vi "unpackWarn.vi"(6 "长度":i32, 7 "数据":u8[](array[numeric]) format="%.0x") -> (2 "告警状态":bool, 3 "告警信息":string)   [LabVIEW 2014]
panel:
  out "告警信息":string
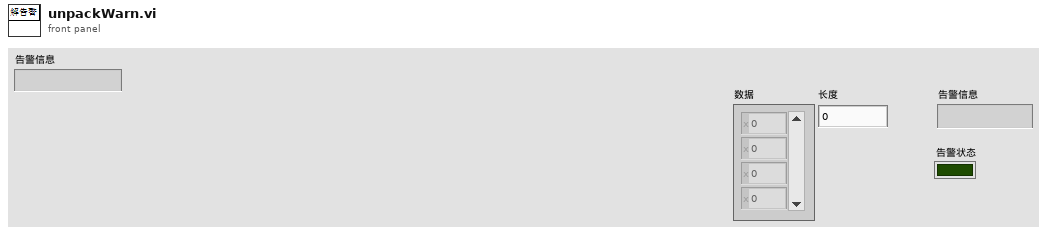
[diagram p1: front panel]
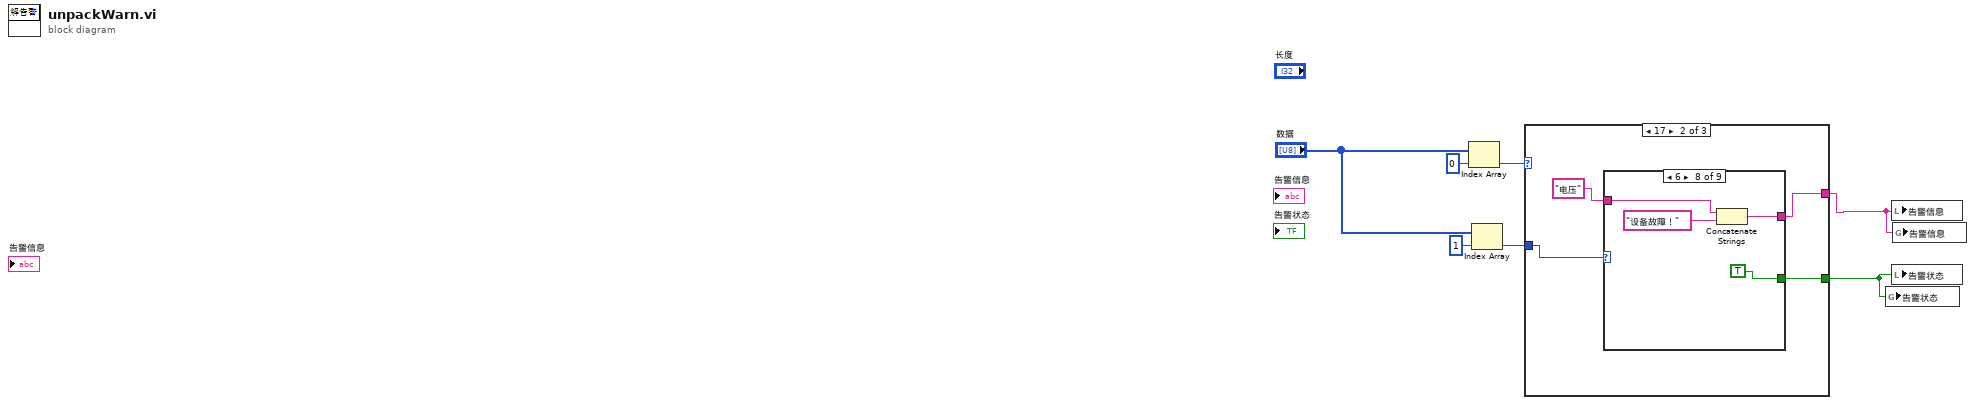
[diagram p0: block diagram]
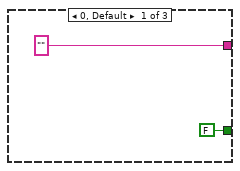
[diagram p2: hidden frame]
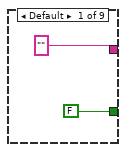
[diagram p3: hidden frame]
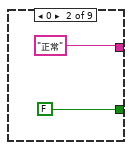
[diagram p4: hidden frame]
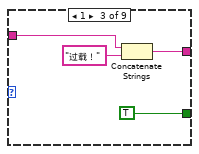
[diagram p5: hidden frame]
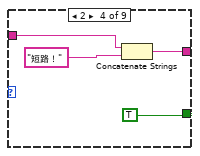
[diagram p6: hidden frame]
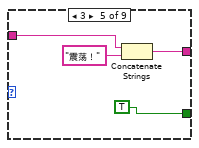
[diagram p7: hidden frame]
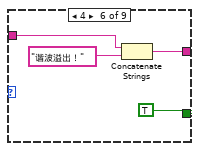
[diagram p8: hidden frame]
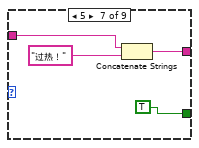
[diagram p9: hidden frame]
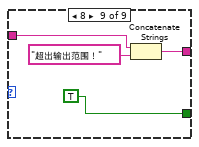
[diagram p10: hidden frame]
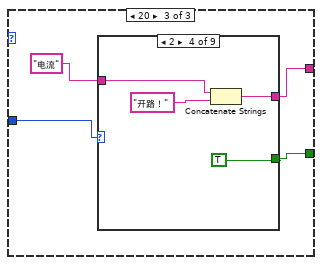
[diagram p11: hidden frame]
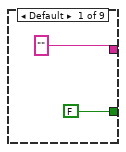
[diagram p12: hidden frame]
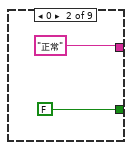
[diagram p13: hidden frame]
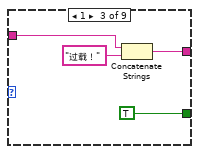
[diagram p14: hidden frame]
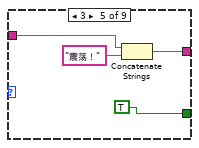
[diagram p15: hidden frame]
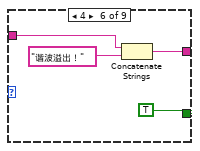
[diagram p16: hidden frame]
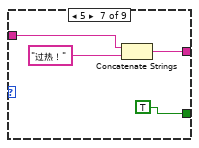
[diagram p17: hidden frame]
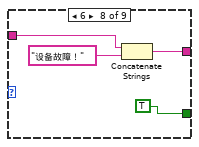
[diagram p18: hidden frame]
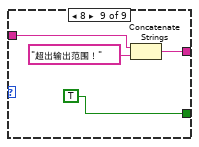
[diagram p19: hidden frame]
diagram:
  n1 = Index Array(array="数据", index=0 ("索引")) -> (element=w6:u8)
  n2 = Index Array(array="数据", index=1 ("索引")) -> (element=w3:u8)
  n3 = case shown="17" w6 {
    tunnel: ["" w11 w47] -> w2
    tunnel: w3 -> [_ w12 w48]
    tunnel: [FALSE ("告警状态") w10 w46] -> w1
    frame 0, Default {
    }
    frame 17 {
      n4 = case shown="6" w12 {
        tunnel: "电压" -> [_ _ w20 w24 w28 w32 w36 w40 w44]
        tunnel: [FALSE ("告警状态") FALSE ("告警状态") TRUE ("告警状态") TRUE ("告警状态") TRUE ("告警状态") TRUE ("告警状态") TRUE ("告警状态") TRUE ("告警状态") TRUE ("告警状态")] -> w10
        tunnel: ["" "正常" w18 w22 w26 w30 w34 w38 w43] -> w11
        frame Default {
        }
        frame 0 {
        }
        frame 1 {
          n5 = Concatenate Strings(w20, "过载！") -> (w18:string)
        }
        frame 2 {
          n6 = Concatenate Strings(w24, "短路！") -> (w22:string)
        }
        frame 3 {
          n7 = Concatenate Strings(w28, "震荡！") -> (w26:string)
        }
        frame 4 {
          n8 = Concatenate Strings(w32, "谐波溢出！") -> (w30:string)
        }
        frame 5 {
          n9 = Concatenate Strings(w36, "过热！") -> (w34:string)
        }
        frame 6 {
          n10 = Concatenate Strings(w40, "设备故障！") -> (w38:string)
        }
        frame 8 {
          n11 = Concatenate Strings(w44, "超出输出范围！") -> (w43:string)
        }
      }
    }
    frame 20 {
      n12 = case shown="2" w48 {
        tunnel: "电流" -> [_ _ w56 w60 w64 w68 w72 w76 w80]
        tunnel: [FALSE ("告警状态") FALSE ("告警状态") TRUE ("告警状态") TRUE ("告警状态") TRUE ("告警状态") TRUE ("告警状态") TRUE ("告警状态") TRUE ("告警状态") TRUE ("告警状态")] -> w46
        tunnel: ["" "正常" w54 w58 w62 w66 w70 w74 w79] -> w47
        frame Default {
        }
        frame 0 {
        }
        frame 1 {
          n13 = Concatenate Strings(w56, "过载！") -> (w54:string)
        }
        frame 2 {
          n14 = Concatenate Strings(w60, "开路！") -> (w58:string)
        }
        frame 3 {
          n15 = Concatenate Strings(w64, "震荡！") -> (w62:string)
        }
        frame 4 {
          n16 = Concatenate Strings(w68, "谐波溢出！") -> (w66:string)
        }
        frame 5 {
          n17 = Concatenate Strings(w72, "过热！") -> (w70:string)
        }
        frame 6 {
          n18 = Concatenate Strings(w76, "设备故障！") -> (w74:string)
        }
        frame 8 {
          n19 = Concatenate Strings(w80, "超出输出范围！") -> (w79:string)
        }
      }
    }
  }
  n20 = global write "系统全局.vi" "告警状态"(w1) -> ()
  n21 = local write "告警信息"(w2) -> ()
  n22 = local write "告警状态"(w1) -> ()
  n23 = global write "系统全局.vi" "告警信息"(w2) -> ()
